vi "Byte Buffer.Read.Typed String.vi"(7 "data type":T1, 8 "error in (no error)":errorcluster, 9 "count":i64, 10 "buffer offset":u64, 11 "Byte Buffer in":refnum<class "Byte Buffer.lvclass">) -> (0 "error out":errorcluster, 1 "string":string, 2 "new buffer offset":u64, 3 "Byte Buffer out":refnum<class "Byte Buffer.lvclass">)   [LabVIEW 2016, in "VeriStand Data.lvlib" / "Byte Buffer.lvclass"]
doc: "Reads <B>count</B> elements of data from the provided <B>Byte Buffer</B> at location <B>buffer offset</B> in the format of the <B>data type</B> specified."
uses:
  Byte Buffer.lvclass
  Typedefs/Typedefs.Data Types.ctl
  Byte Buffer.lvclass/Byte Buffer.ctl
  Byte Buffer.Get Buffer Size.vi
  Memory Management/Memory Management.MoveByteBlock.Write (String).vi
  Byte Buffer.Get Buffer Pointer.vi
  Utilities/Utilities.Sizeof.Scalar.vi
  Memory Management/Memory Management.Handle Return.vi
  VeriStand Data.lvlib
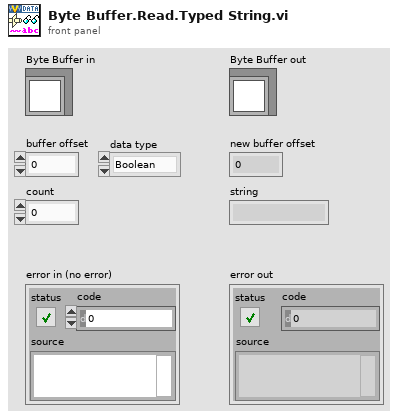
[diagram p1: front panel]
types:
  T1 = typedef "VeriStand Data.lvlib/Typedefs.Data Types.ctl" = enum16{"Boolean", "Single", "Double", "I8", "I16", "I32", "I64", "U8", "U16", "U32", "U64"}
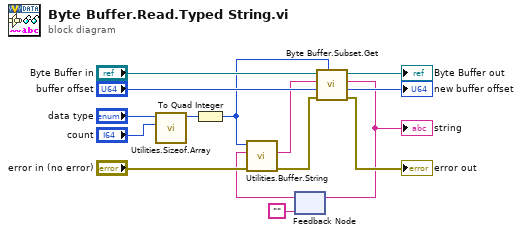
[diagram p0: block diagram]
diagram:
  n1 = call "Utilities.Sizeof.Array.vi"("count"="count", "data type"="data type") -> ("size"=w10:u64)  [unwired: 9 in]
  n2 = To Quad Integer(1:w10) -> (0:w3:i64)
  n3 = feedback #1("") -> (w2:string)
  n4 = call "Utilities.Buffer.String.vi"("error in (no error)"="error in (no error)", "buffer in"=w2, "minimum size"=w3) -> ("error out"=w5:errorcluster, "buffer out"=w4:string)  [unwired: 7 in]
  n5 = call "Byte Buffer.Subset.Get.vi"("length (-1: rest)"=w3, "error in (no error)"=w5, "offset (0)"="buffer offset", "allocated string in"=w4, "Byte Buffer in"="Byte Buffer in") -> ("error out"=→"error out":errorcluster, "new buffer offset"=→"new buffer offset":u64, "string out"=w7:string, "Byte Buffer out"=→"Byte Buffer out":refnum<class "Byte Buffer.lvclass">)  [unwired: 3 in]
  "string" <- w7
  n6 = feedback-in #1(w7) -> ()
